vi "LED Spike.vi"(9 "ON/OFF":bool, 11 "State":enum16{"Open", "Run", "End"}(ring)=enum."Run") -> ()   [LabVIEW 2013]
uses:
  <vilib>/Rock Robotics/SystemInterfaces/DIO/FPGA_DIORelayChannel.ctl
  <vilib>/Rock Robotics/SystemInterfaces/Typedef/FPGA_TypedefDigitalModule.ctl
  <vilib>/Rock Robotics/WPI/Relay/WPI_RelayDirection.ctl
  <vilib>/Rock Robotics/WPI/Relay/WPI_RelayValue.ctl
panel:
  in  "DIO Module":T1
  in  "RelayChannel":T2
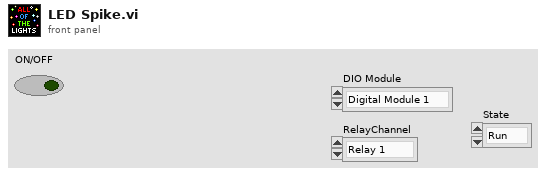
[diagram p1: front panel]
types:
  T1 = typedef "FPGA_TypedefDigitalModule.ctl" = enum16{"Digital Module 1", "Digital Module 2"}
  T2 = typedef "FPGA_DIORelayChannel.ctl" = enum8{"Relay 1", "Relay 2", "Relay 3", "Relay 4", "Relay 5", "Relay 6", "Relay 7", "Relay 8", "Invalid"}
  T3 = typedef "WPI_RelayDirection.ctl" = enum16{"Both directions", "Forward only", "Reverse only"}
  T4 = typedef "WPI_RelayValue.ctl" = enum16{"Off", "On", "Forward", "Reverse"}
  T5 = typedef "WPI_RelayDevRef.ctl" = cluster{"DevStatus":errorcluster, "Relay Channel":T2, "Digital Module":T1, "Relay Direction":T3}
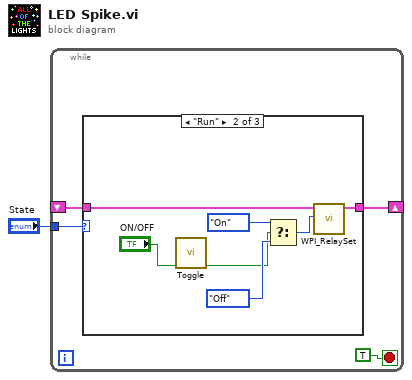
[diagram p0: block diagram]
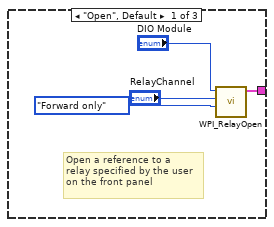
[diagram p2: hidden frame]
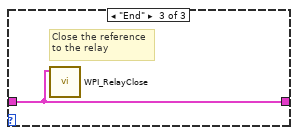
[diagram p3: hidden frame]
diagram:
  n1 = while {
    tunnel: "State" -> [w4]
    shift-right: [w3] -> _
    shift-left: _ -> [w2]
    stop <- TRUE stop-if-true
    n2 = case shown="\"Run\"" w4 {
      tunnel: [w6 w15 w17] -> w3
      tunnel: w2 -> [_ w16 w17]
      frame "Open", Default {
        # "Open a reference to a \nrelay specified by the user\non the front panel"
        n3 = call <vilib>:"WPI_RelayOpen.vi"("Relay Direction"=WPI_RelayDirection."Forward only" ("RelayDirection"), "Relay Channel"="RelayChannel", "Digital Module (Module 1)"="DIO Module") -> ("RelayDevRef"=w6:T5)  [unwired: 1 in, 7 out]
      }
      frame "Run" {
        n4 = call "Toggle.vi"("Input"="ON/OFF") -> ("Latched"=w10:bool)  [unwired: 10 in]
        n5 = Select(t=WPI_RelayValue."On" ("RelayValue"), s=w10, f=WPI_RelayValue."Off" ("RelayValue")) -> (s? t:f=w12:T4)
        n6 = call <vilib>:"WPI_RelaySet.vi"("RelayValue"=w12, "RelayDevRef"=w16) -> ("RelayDevRef"=w15:T5)  [unwired: 1 in, 8 out]
      }
      frame "End" {
        # "Close the reference\nto the relay"
        n7 = call <vilib>:"WPI_RelayClose.vi"("RelayDevRef"=w17) -> ()  [unwired: 1 in, 10 out]
      }
    }
  }
